vi "Edit_String_Options_list.vi"(2 "Channel Name":string, 3 "String array":string[](array[string])) -> (0 "New Selection Index":i32, 1 "String array Out":string[](array[string]))   [LabVIEW 2018]
uses:
  Controls/ok_button.ctl
panel:
  in  "Menu Strings":string[][](table)
  out "Meassage":string
  in  "OK":T1
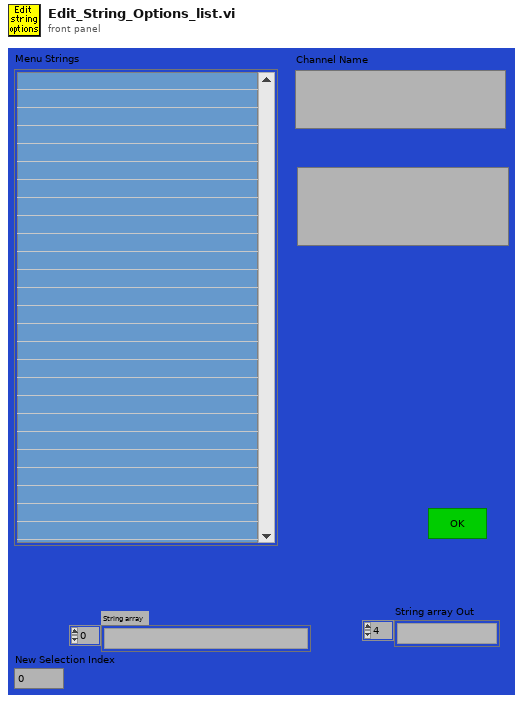
[diagram p1: front panel]
types:
  T1 = typedef "ok_button.ctl" = bool
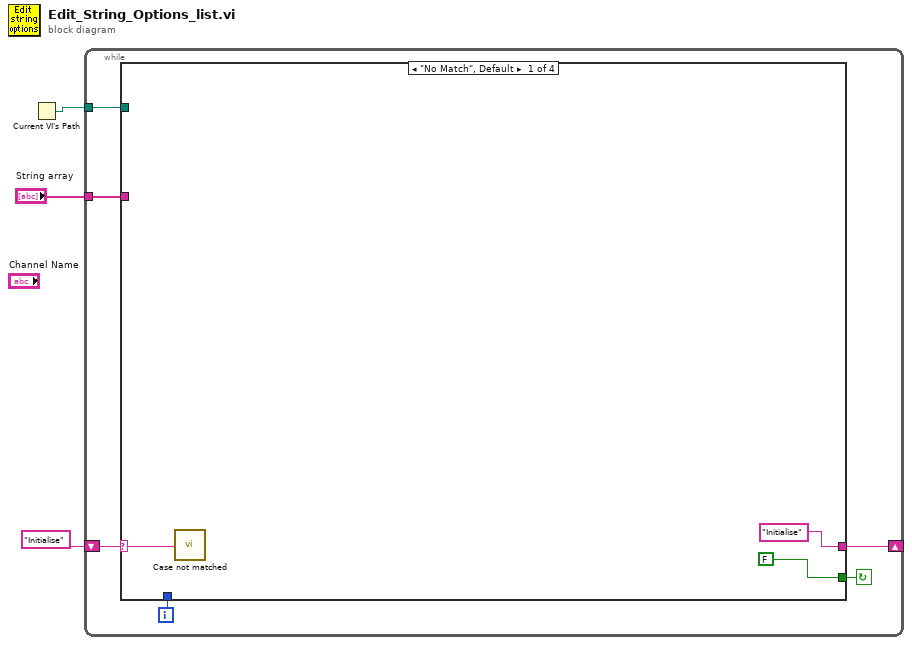
[diagram p0: block diagram]
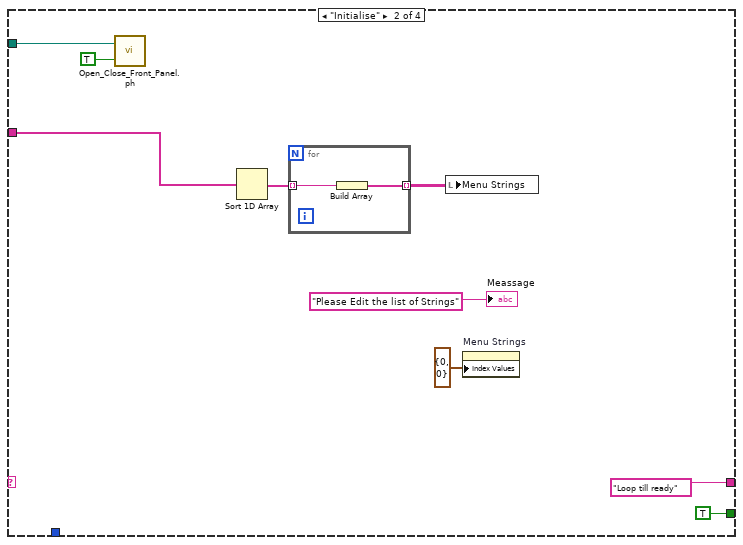
[diagram p2: hidden frame]
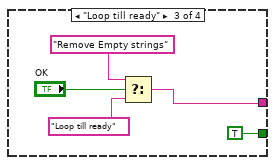
[diagram p3: hidden frame]
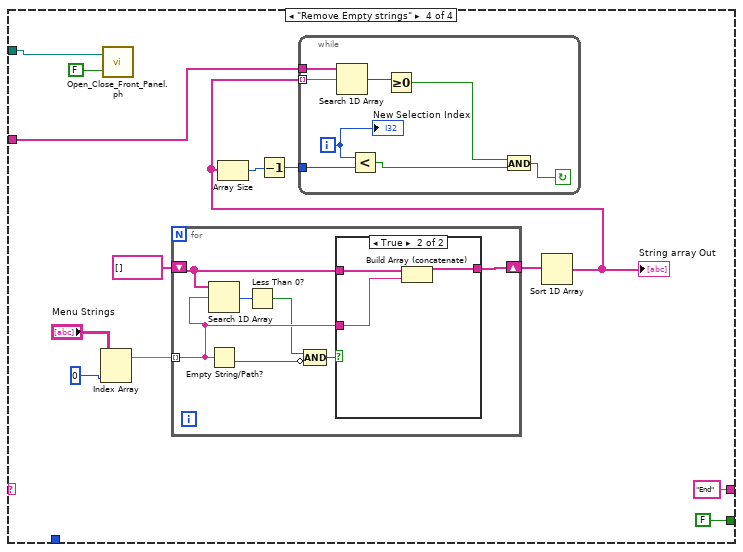
[diagram p4: hidden frame]
diagram:
  n1 = Current VI's Path() -> (path=w2:path)
  n2 = while {
    shift-left: "Initialise" -> [w7]
    shift-right: [w8] -> _
    tunnel: w2 -> [w5]
    tunnel: "String array" -> [w4]
    i -> [w6]
    stop <- w9 continue-if-true
    n3 = case shown="\"No Match\", Default" w7 {
      selector: w7 -> [w10 _ _ _]
      tunnel: [FALSE TRUE TRUE FALSE] -> w9
      tunnel: ["Initialise" "Loop till ready" w25 "End"] -> w8
      tunnel: w6 -> [_ _ _ _]
      tunnel: w5 -> [_ w15 _ w33]
      tunnel: w4 -> [_ w13 _ w32]
      frame "No Match", Default {
        n4 = call "Case not matched.vi"("Case Name not Matched"=w10) -> ()
      }
      frame "Initialise" {
        n5 = call "Open_Close_Front_Panel.ph.vi"("Front Panel Window:Open"=TRUE, "VI path"=w15) -> ()  [unwired: 2 out]
        n6 = Sort 1D Array(array=w13) -> (sorted array=w17:string[])
        n7 = for {
          tunnel: [w23] -> w16 mode=indexing
          tunnel: w17 -> [w22] mode=indexing
          n8 = Build Array(w22) -> (w23:string[])
        }
        n9 = local write "Menu Strings"(w16) -> ()
        n10 = property on="Menu Strings" class="Tbl (strict)"("Index Values"=cluster{u32, u32} {0, 0} ("Write Attribute")) -> ()  [unwired: 2 in, 2 out]
        "Meassage" <- "Please Edit the list of Strings" ("String")
      }
      frame "Loop till ready" {
        n11 = Select(t="Remove Empty strings", s="OK", f="Loop till ready") -> (s? t:f=w25:string)
      }
      frame "Remove Empty strings" {
        n12 = Index Array(array="Menu Strings", index (col)=0 ("Index")) -> (element=w36:string[])  [unwired: 1 in]
        n13 = call "Open_Close_Front_Panel.ph.vi"("Front Panel Window:Open"=FALSE, "VI path"=w33) -> ()  [unwired: 2 out]
        n14 = for {
          shift-right: [w56] -> w35
          shift-left: string[] [] -> [w55]
          tunnel: w36 -> [w54] mode=indexing
          n15 = Search 1D Array(1D array=w55, element=w54) -> (index of element=w53:i32)  [unwired: 1 out]
          n16 = Empty String/Path?(string/path=w54) -> (empty?=w51:bool)
          n17 = Less Than 0?(x=w53) -> (x < 0?=w52:bool)
          n18 = Compound Arithmetic op=AND(w52, invert w51) -> (w50:bool)
          n19 = case shown="True" w50 {
            tunnel: w55 -> [w57 w60]
            tunnel: [w57 w59] -> w56
            tunnel: w54 -> [_ w58]
            frame False {
            }
            frame True {
              n20 = Build Array (concatenate)(w60, w58) -> (w59:string[])
            }
          }
        }
        n21 = Sort 1D Array(array=w35) -> (sorted array=w31:string[])
        "String array Out" <- w31
        n22 = Array Size(array=w31) -> (size(s)=w30:i32)
        n23 = Decrement(x=w30) -> (x-1=w29:i32)
        n24 = while {
          tunnel: w31 -> [w49] mode=indexing
          tunnel: w32 -> [w48]
          tunnel: w29 -> [w46]
          i -> [w47]
          stop <- w44 continue-if-true
          n25 = Search 1D Array(1D array=w48, element=w49) -> (index of element=w43:i32)  [unwired: 1 out]
          n26 = Less?(x=w47, y=w46) -> (x < y?=w45:bool)
          n27 = Greater Or Equal To 0?(x=w43) -> (x >= 0?=w42:bool)
          n28 = And(x=w42, y=w45) -> (x .and. y?=w44:bool)
          "New Selection Index" <- w47
        }
      }
    }
  }
